vi "FPGA Time Tag.vi"(7 "runs":i32, 8 "error in (no error)":errorcluster, 9 "fileName":string, 10 "fpgaCommand":u8, 11 "saveClicks":bool) -> (0 "error out":errorcluster, 1 "fileName out":string, 3 "function return":i32, 4 "stats":i64[](array[numeric]))   [LabVIEW 2015, in "Stats.lvlib"]
doc: "Get timestamped clicks from four channels using a Xylo-EM FPGA board.\n\nLIBRARY_API int FPGA_TimeTag(bool saveClicks, unsigned char fpgaCommand,char* fileName, int* stats, int runs);\nLIBRARY_API int FPGA_TimeTag(bool saveClicks, unsigned char fpgaCommand, char* fileName, __int64* stats, int runs);"
uses:
  Stats.lvlib
  Stats/Release/x64/Stats.dll
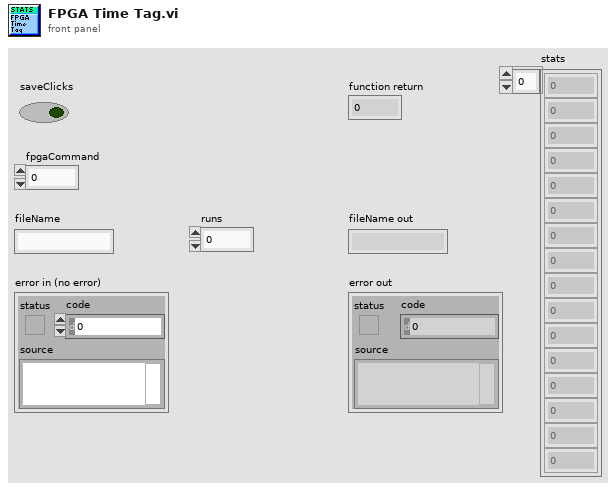
[diagram p1: front panel]
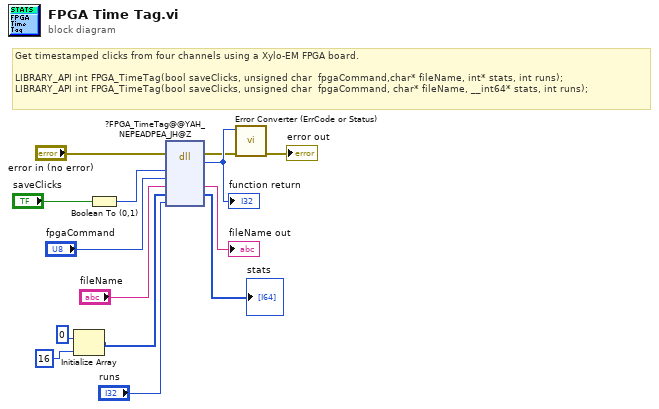
[diagram p0: block diagram]
diagram:
  # "Get timestamped clicks from four channels using a Xylo-EM FPGA board.\n\nLIBRARY_API int FPGA_TimeTag(bool saveClicks, unsigned char  fpgaCommand,char* fileName, int* stats, int runs);\nLIBRARY_API int FPGA_TimeTag(bool saveClicks, unsigned char  fpgaCommand, char* fileName, __int64* stats, int runs);"
  n1 = Initialize Array(0, 16) -> (w1:i32[])
  n2 = Boolean To (0,1)(Boolean="saveClicks") -> (0, 1=w12:i16)
  n3 = dll-call lib="C:/FPGA_Lauren/Stats_NIST_file/Stats/Release/x64/Stats.*" fn="?FPGA_TimeTag@@YAH_NEPEADPEA_JH@Z"(error in="error in (no error)", "saveClicks"=w12, "fpgaCommand"="fpgaCommand", "fileName"="fileName", "stats"=w1, "runs"="runs") -> (error out=w6:errorcluster, "return type"=w14:i32, "fileName"=→"fileName out":string, "stats"=→"stats":i64[])  [unwired: 5 in, 1 out]
  "function return" <- w14
  n4 = call "Error Converter (ErrCode or Status).vi"("error in (no error)"=w6, "error code"=w14) -> ("error out"=→"error out":errorcluster)  [unwired: 9 in]
